vi "Configure.vi"(8 "error in (no error)":errorcluster, 11 "Mouse in":refnum<class "Mouse.lvclass">) -> (0 "error out":errorcluster, 3 "Mouse out":refnum<class "Mouse.lvclass">)   [LabVIEW 2020, in "Maze.lvlib" / "Mouse.lvclass"]
doc: "Configure can optionally be overridden to allow changing parameters for the mouse's navigation algorithms. This is useful for developers to more rapidly test different parameters of their algorithm without needing to rebuild their mouse to set new default values. However for the final submission this will not be used so make sure once optimal parameters are discovered using this VI that they are set as default values for the mouse."
uses:
  Mouse.lvclass
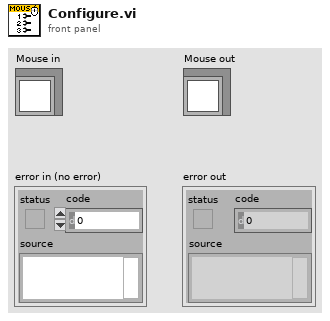
[diagram p1: front panel]
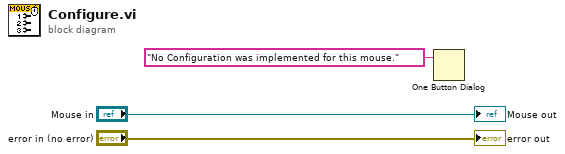
[diagram p0: block diagram]
diagram:
  n1 = One Button Dialog(message="No Configuration was implemented for this mouse.") -> ()  [unwired: 1 in, 1 out]
  "error out" <- "error in (no error)"
  "Mouse out" <- "Mouse in"
